vi "Unsubscribe from Group (SubVI).vi"(8 "error in (no error)":errorcluster, 9 "group":string, 11 "first_name":string) -> (0 "error out":errorcluster)   [LabVIEW 2020, in "Notification.lvlib"]
uses:
  Notification.lvlib
  <vilib>/Utility/config.llb/NI_LVConfig.lvlib
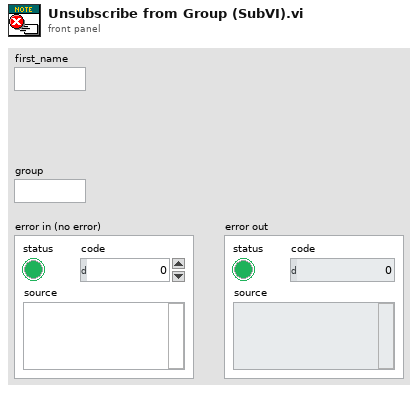
[diagram p1: front panel]
types:
  T1 = typedef "NI_LVConfig.lvlib/Config Data RefNum.ctl" = refnum<k1>
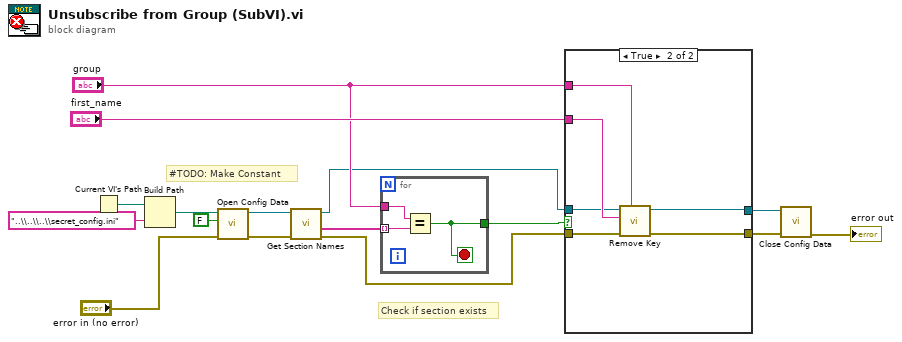
[diagram p0: block diagram]
diagram:
  # "#TODO: Make Constant"
  # "Check if section exists"
  n1 = Current VI's Path() -> (path=w4:path)
  n2 = Build Path(base path=w4, name or relative path="..\\..\\..\\secret_config.ini") -> (appended path=w2:path)
  n3 = call <vilib>:"Open Config Data.vi"("error in (no error)"="error in (no error)", "create file if necessary (T)"=FALSE, "configuration file path"=w2) -> ("error out"=w14:errorcluster, "refnum"=w13:T1)  [unwired: 6 in, 1 out]
  n4 = call <vilib>:"Get Section Names.vi"("error in (no error)"=w14, "refnum"=w13) -> ("error out"=w9:errorcluster, "section names"=w11:string[], "refnum out"=w6:T1)  [unwired: 7 in]
  n5 = for {
    tunnel: "group" -> [w18]
    tunnel: w11 -> [w19] mode=indexing
    tunnel: [w17] -> w10
    stop <- w17 stop-if-true
    n6 = Equal?(x=w18, y=w19) -> (x = y?=w17:bool)
  }
  n7 = case shown="True" w10 {
    tunnel: "first_name" -> [_ w27]
    tunnel: "group" -> [_ w26]
    tunnel: w9 -> [w21 w25]
    tunnel: [w21 w22] -> w8
    tunnel: [w20 w23] -> w7
    tunnel: w6 -> [w20 w24]
    frame False {
    }
    frame True {
      n8 = call <vilib>:"Remove Key.vi"("section"=w26, "error in (no error)"=w25, "key"=w27, "refnum"=w24) -> ("error out"=w22:errorcluster, "refnum out"=w23:T1)  [unwired: 5 in, 1 out]
    }
  }
  n9 = call <vilib>:"Close Config Data.vi"("error in (no error)"=w8, "refnum"=w7) -> ("error out"=→"error out":errorcluster)  [unwired: 8 in, 1 out]
